vi "Create DateTime String.vi"(8 "error in (no error)":errorcluster, 11 "Report in":refnum<class "Report.lvclass">) -> (0 "error out":errorcluster, 3 "Report out":refnum<class "Report.lvclass">)   [LabVIEW 2023, in "Report.lvlib" / "Report.lvclass"]
uses:
  Report.lvclass
  Report.lvclass/Report.ctl
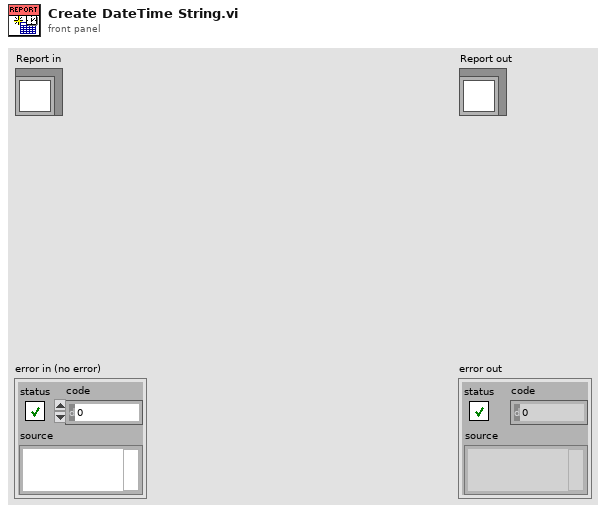
[diagram p1: front panel]
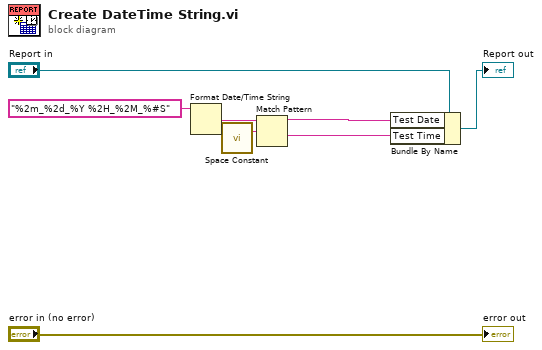
[diagram p0: block diagram]
diagram:
  n1 = Format Date/Time String(time format string (%c)="%2m_%2d_%Y %2H_%2M_%#S") -> (date/time string=w7:string)  [unwired: 2 in]
  n2 = call <vilib>:"Space Constant.vi"() -> ("String"=w6:string)
  n3 = Match Pattern(string=w7, regular expression=w6) -> (before substring=w4:string, after substring=w3:string)  [unwired: 1 in, 2 out]
  n4 = Bundle By Name(cluster="Report in", "Test Date"=w4, "Test Time"=w3) -> (→"Report out":refnum<class "Report.lvclass">)
  "error out" <- "error in (no error)"
